vi "determine_gain.vi"(8 "error in (no error)":errorcluster, 11 "VISA resource name":refnum<visa-resource-name>) -> (0 "error out":errorcluster, 3 "VISA resource name out":refnum<visa-resource-name>)   [LabVIEW 2018]
uses:
  <instrlib>/Stanford Research 830/Public/Data/Read (1 Parameter).vi
  <instrlib>/Stanford Research 830/Stanford Research 830.lvlib
panel:
  in  "Parameter (1: X)":u16(ring)=3 items=["X"=1, "Y"=2, "R"=3, "Theta"=4, "Channel 1"=5, "Channel 2"=6, "Aux In 1"=7, "Aux In 2"=8, "Aux In 3"=9, "Aux In 4"=10]
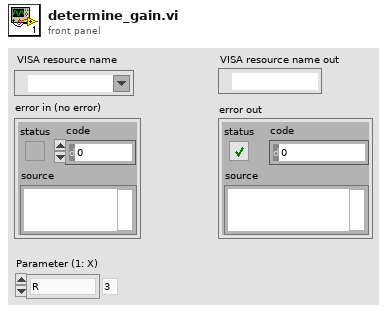
[diagram p1: front panel]
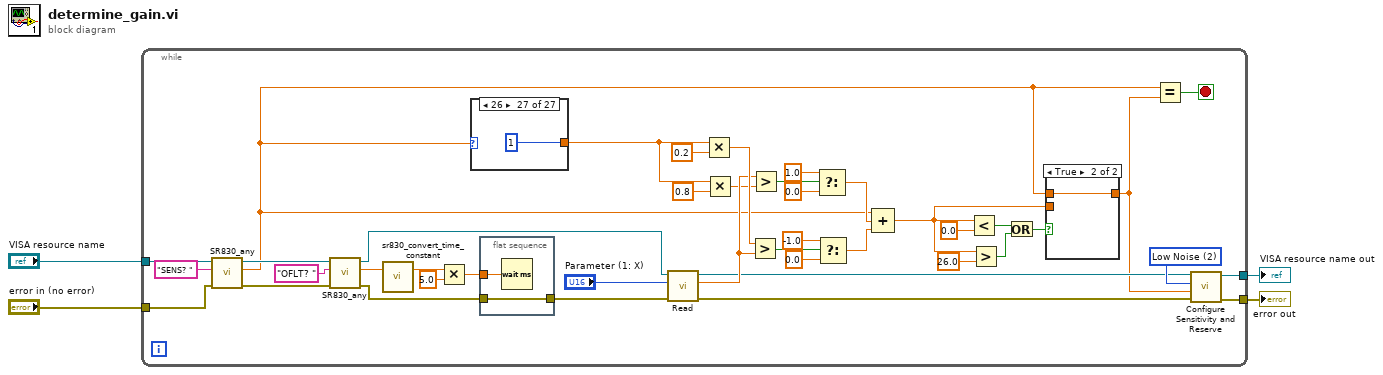
[diagram p0: block diagram]
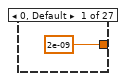
[diagram p3: hidden frame]
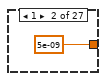
[diagram p4: hidden frame]
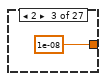
[diagram p5: hidden frame]
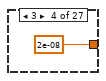
[diagram p6: hidden frame]
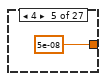
[diagram p7: hidden frame]
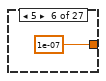
[diagram p8: hidden frame]
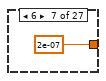
[diagram p9: hidden frame]
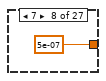
[diagram p10: hidden frame]
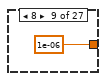
[diagram p11: hidden frame]
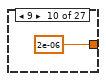
[diagram p12: hidden frame]
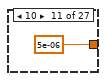
[diagram p13: hidden frame]
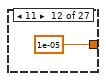
[diagram p14: hidden frame]
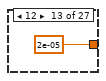
[diagram p15: hidden frame]
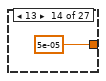
[diagram p16: hidden frame]
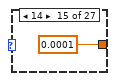
[diagram p17: hidden frame]
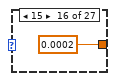
[diagram p18: hidden frame]
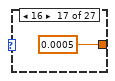
[diagram p19: hidden frame]
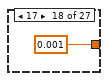
[diagram p20: hidden frame]
diagram:
  n1 = while {
    tunnel: "VISA resource name" -> [w38]
    tunnel: "error in (no error)" -> [w32]
    tunnel: [w6] -> w1
    tunnel: [w5] -> w2
    stop <- w15 stop-if-true
    w45 = i16 2 items=["Auto Reserve"=-1, "High Reserve"=0, "Normal"=1, "Low Noise"=2] ("Dynamic Reserve (-1: Auto Reserve)")
    n2 = call "SR830_any.vi"("error in (no error)"=w32, "initial string"="SENS? ", "VISA resource name"=w38) -> ("error out"=w36:errorcluster, "Measurement"=w9:dbl, "VISA resource name out"=w37:refnum<visa-resource-name>)  [unwired: 6 in]
    n3 = call "SR830_any.vi"("error in (no error)"=w36, "initial string"="OFLT? ", "VISA resource name"=w37) -> ("error out"=w35:errorcluster, "Measurement"=w40:dbl, "VISA resource name out"=w33:refnum<visa-resource-name>)  [unwired: 6 in]
    n4 = call "sr830_convert_time_constant.vi"("Time constant code"=w40) -> ("time constant  in ms"=w43:dbl)  [unwired: 2 in]
    n5 = Multiply(x=w43, y=5.0) -> (x*y=w39:dbl)
    n6 = case shown="26" w9 {
      tunnel: [2e-09 5e-09 1e-08 2e-08 5e-08 1e-07 2e-07 5e-07 1e-06 2e-06 5e-06 1e-05 2e-05 5e-05 0.0001 0.0002 0.0005 0.001 0.002 0.005 0.01 0.02 0.05 0.1 0.2 0.5 1] -> w28
      frame 0, Default {
      }
      frame 1 {
      }
      frame 2 {
      }
      frame 3 {
      }
      frame 4 {
      }
      frame 5 {
      }
      frame 6 {
      }
      frame 7 {
      }
      frame 8 {
      }
      frame 9 {
      }
      frame 10 {
      }
      frame 11 {
      }
      frame 12 {
      }
      frame 13 {
      }
      frame 14 {
      }
      frame 15 {
      }
      frame 16 {
      }
      frame 17 {
      }
      frame 18 {
      }
      frame 19 {
      }
      frame 20 {
      }
      frame 21 {
      }
      frame 22 {
      }
      frame 23 {
      }
      frame 24 {
      }
      frame 25 {
      }
      frame 26 {
      }
    }
    n7 = flat-sequence {
      tunnel: w39 -> [w77]
      tunnel: [w76] -> w34
      tunnel: w35 -> [w76]
      frame #0 {
        n8 = Wait (ms)(milliseconds to wait=w77) -> ()  [unwired: 1 out]
      }
    }
    n9 = call-poly <instrlib>:"Read.vi"("error in (no error)"=w34, "Parameter (1: X)"="Parameter (1: X)", "VISA resource name"=w33) -> ("error out"=w17:errorcluster, "Measurement"=w27:dbl, "VISA resource name out"=w16:refnum<visa-resource-name>)  [unwired: 6 in]
    n10 = Multiply(x=w28, y=0.2) -> (x*y=w30:dbl)
    n11 = Multiply(x=w28, y=0.8) -> (x*y=w26:dbl)
    n12 = Greater?(x=w30, y=w27) -> (0:w20:bool)
    n13 = Greater?(x=w27, y=w26) -> (0:w25:bool)
    n14 = Select(t=1.0, s=w25, f=0.0) -> (s? t:f=w18:dbl)
    n15 = Select(t=-1.0, s=w20, f=0.0) -> (s? t:f=w19:dbl)
    n16 = Compound Arithmetic op=ADD(w9, w18, w19) -> (w7:dbl)
    n17 = Less?(x=w7, y=0.0) -> (x < y?=w12:bool)
    n18 = Greater?(x=w7, y=26.0) -> (0:w11:bool)
    n19 = Or(x=w12, y=w11) -> (x .or. y?=w10:bool)
    n20 = case shown="True" w10 {
      tunnel: w9 -> [_ w48]
      tunnel: [w47 w48] -> w8
      tunnel: w7 -> [w47 _]
      frame False {
      }
      frame True {
      }
    }
    n21 = Equal?(x=w9, y=w8) -> (x = y?=w15:bool)
    n22 = call <instrlib>:"Configure Sensitivity and Reserve.vi"("error in (no error)"=w17, "Sensitivity (-1: Auto gain)"=w8, "Dynamic Reserve (-1: Auto Reserve)"=w45, "VISA resource name"=w16) -> ("error out"=w6:errorcluster, "VISA resource name out"=w5:refnum<visa-resource-name>)  [unwired: 6 in]
  }
  "VISA resource name out" <- w2
  "error out" <- w1
